vi "UI_Get Focus Index.vi"(8 "Error":errorcluster, 11 "Ref String  Array":refnum<vi>[](array[refnum])) -> (0 "Error Out":errorcluster, 3 "Focus Index Out":i32)   [LabVIEW 2009]
doc: "Retrieves the index of the string control that has focus"
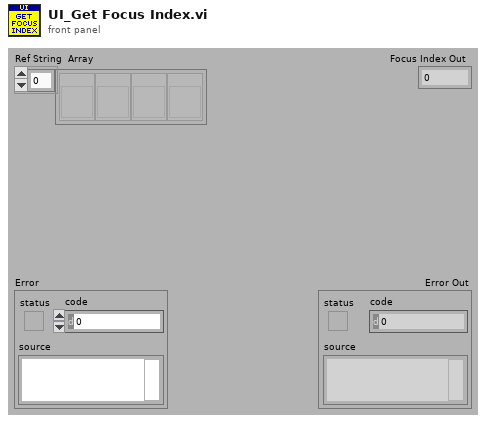
[diagram p1: front panel]
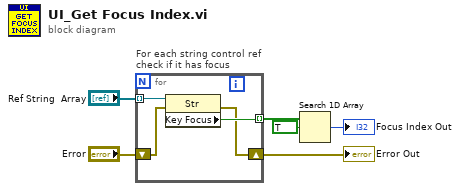
[diagram p0: block diagram]
diagram:
  n1 = for "For each string control ref\ncheck if it has focus" {
    tunnel: "Ref String  Array" -> [w10] mode=indexing
    tunnel: [w9] -> w3 mode=indexing
    shift-right: [w8] -> w2
    shift-left: "Error" -> [w7]
    n2 = property class="Str"(reference=w10, error in=w7) -> (error out=w8:errorcluster, "Key Focus"=w9:bool)  [unwired: 1 out]
  }
  "Error Out" <- w2
  n3 = Search 1D Array(1D array=w3, element=TRUE) -> (index of element=→"Focus Index Out":i32)  [unwired: 1 in]
